vi "Wake up HL.vi"(6 "wait for reply (T)":bool=TRUE, 8 "error in":errorcluster, 10 "Acquisition data":T1, 11 "Module ID":i32=-1) -> (0 "error out":errorcluster, 1 "timed out?":bool, 3 "Data out":variant)   [LabVIEW 2020, in "NI DAQ.lvlib"]
doc: "Request to wake the helper loop to continuously read\\acquire from the specified task at a rate detemined by the timeout. Returns data as a variant.\n_____\nCreated using DQMH Event Scripter 6.1.0.128."
uses:
  NI DAQ.lvlib
  Support/Continuous aquisition params.ctl
  Support/Task list.ctl
  Wake up HL Argument--cluster.ctl
  Wake up HL (Reply Payload)--cluster.ctl
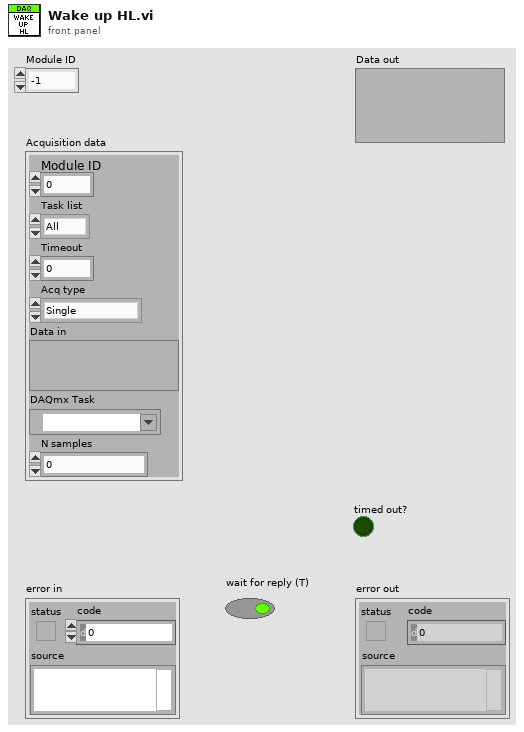
[diagram p1: front panel]
types:
  T1 = typedef "NI DAQ.lvlib/Continuous aquisition params.ctl" = cluster{"Module ID":i32, "Task list":T2, "Timeout":i32, "Acq type":enum16{"Single", "Multiple"}, "Data in":variant, "DAQmx Task":refnum<k21>, "N samples":i32}
  T2 = typedef "NI DAQ.lvlib/Task list.ctl" = enum16{"All", "DO task", "DI task", "AO task", "AI task"}
  T3 = typedef "NI DAQ.lvlib/Wake up HL Argument--cluster.ctl" = cluster{"Module ID":i32, "Wait Notifier":refnum<notifier>, "wait for reply":bool, "Acquisition data":T1}
  T4 = typedef "NI DAQ.lvlib/Request Events--cluster.ctl" = cluster{"Stop Module":refnum<user-event>, "Show Panel":refnum<user-event>, "Hide Panel":refnum<user-event>, "Show Diagram":refnum<user-event>, "Get Module Execution Status":refnum<user-event>, "Set device ID":refnum<user-event>, "Get channel list":refnum<user-event>, "Create DO task":refnum<user-event>, "Start task":refnum<user-event>, "Stop task":refnum<user-event>, "Write DO":refnum<user-event>, "Create DI channel":refnum<user-event>, "Read DI":refnum<user-event>, "Get task ref":refnum<user-event>, "Wake up HL":refnum<user-event>, "Sleep HL":refnum<user-event>, "Create AI channel":refnum<user-event>, "Read AI":refnum<user-event>, "Create AO channel":refnum<user-event>, "Write AO":refnum<user-event>, "Validate connection":refnum<user-event>, "Start continous acquisition":refnum<user-event>, "Stop continuous acquisition":refnum<user-event>}
  T5 = typedef "NI DAQ.lvlib/Wake up HL (Reply Payload)--cluster.ctl" = cluster{"data":variant, "error":errorcluster}
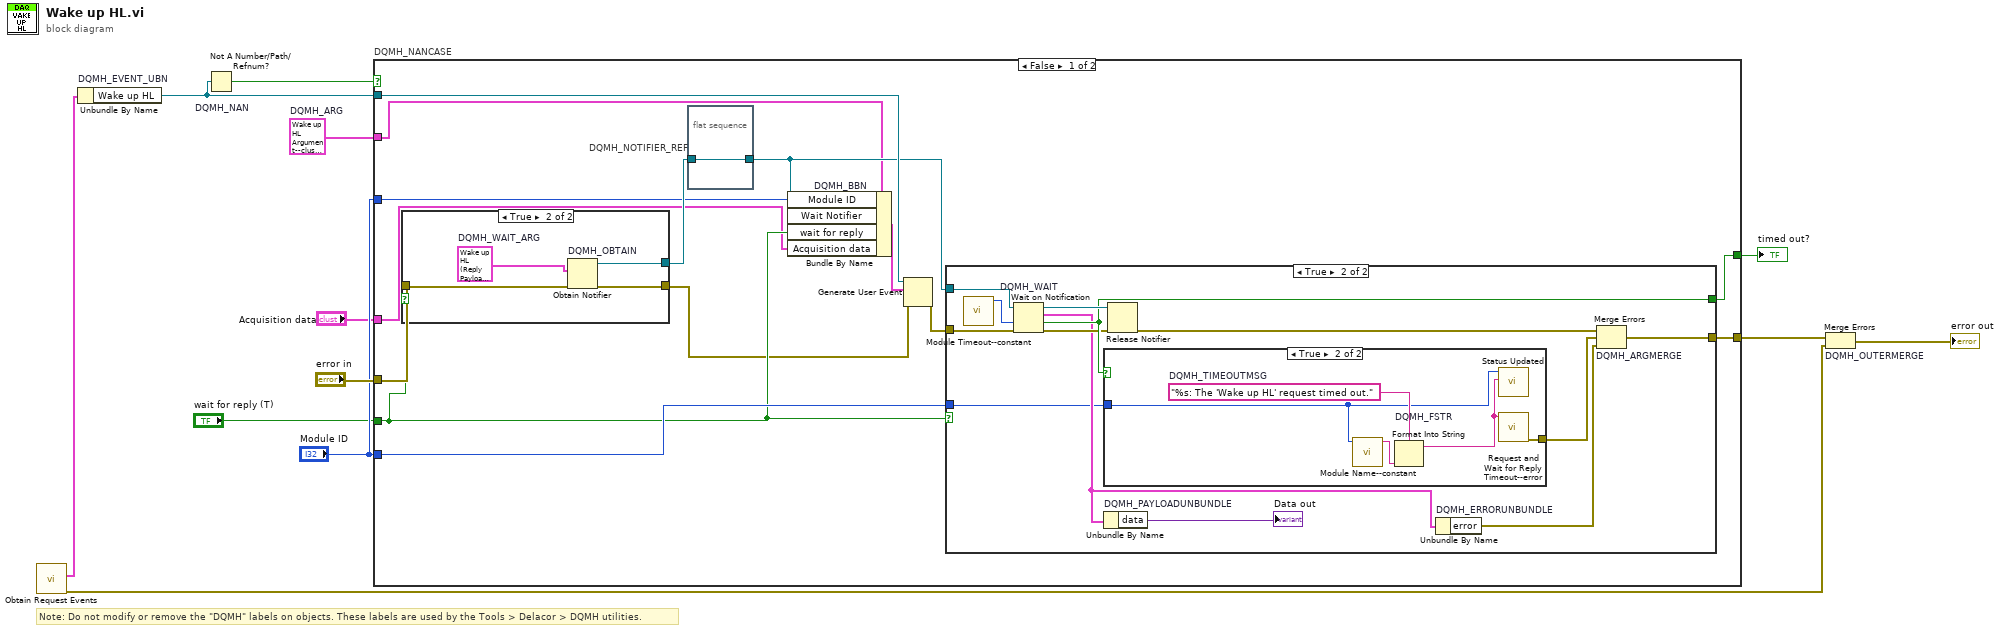
[diagram p0: block diagram]
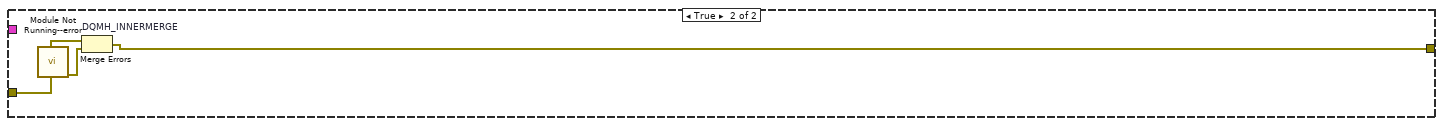
[diagram p5: hidden frame]
diagram:
  w6 = T3 {"Module ID"=-1, "Wait Notifier"=refnum, "wait for reply"=FALSE, "Acquisition data"={"Module ID"=0, "Task list"=enum."DO task", "Timeout"=0, "Acq type"=enum."Single", "Data in"=variant, "DAQmx Task"="", "N samples"=0}}  # DQMH_ARG
  # "Note: Do not modify or remove the \"DQMH\" labels on objects. These labels are used by the Tools > Delacor > DQMH utilities."
  n1 = call "Obtain Request Events.vi"() -> ("error out"=w3:errorcluster, "NI DAQ Request Events"=w2:T4)  [unwired: 10 in]
  n2 = Unbundle By Name "DQMH_EVENT_UBN"(w2) -> ("Wake up HL"=w10:refnum<user-event>)
  n3 = Not A Number/Path/Refnum? "DQMH_NAN"(number/path/refnum=w10) -> (NaN/Path/Refnum?=w9:bool)
  n4 = case "DQMH_NANCASE" shown="False" w9 {
    tunnel: "error in" -> [w26 w54]
    tunnel: w10 -> [w24 _]
    tunnel: [w22 w53] -> w7
    tunnel: [w23 _] -> w8
    tunnel: w6 -> [w18 _]
    tunnel: "Module ID" -> [w17 _]
    tunnel: "Module ID" -> [w16 _]
    tunnel: "wait for reply (T)" -> [w15 _]
    tunnel: "Acquisition data" -> [w13 _]
    frame False {
      n5 = case shown="True" w15 {
        tunnel: w26 -> [w47 w51]
        tunnel: [w47 w50] -> w14
        tunnel: [_ w48] -> w20
        frame False {
        }
        frame True {
          w49 = T5 {"data"=variant, "error"={"status"=FALSE, "code"=0, "source"=""}}  # DQMH_WAIT_ARG
          n6 = Obtain Notifier "DQMH_OBTAIN"(notification data type=w49, error in (no error)=w51) -> (notifier out=w48:refnum<notifier>, error out=w50:errorcluster)  [unwired: 2 in, 1 out]
        }
      }
      n7 = flat-sequence "DQMH_NOTIFIER_REF" {
        tunnel: w20 -> [w27]
        tunnel: [w27] -> w19
        frame #0 {
        }
      }
      n8 = Bundle By Name "DQMH_BBN"(cluster=w18, "Module ID"=w17, "Wait Notifier"=w19, "wait for reply"=w15, "Acquisition data"=w13) -> (w21:T3)
      n9 = Generate User Event(user event=w24, event data cluster=w21, error in=w14) -> (error out=w25:errorcluster)  [unwired: 1 in, 1 out]
      n10 = case shown="True" w15 {
        tunnel: w25 -> [w28 w41]
        tunnel: w19 -> [_ w40]
        tunnel: [_ w38] -> w23
        tunnel: [w28 w37] -> w22
        tunnel: w16 -> [_ w29]
        frame False {
        }
        frame True {
          n11 = call "Module Timeout--constant.vi"() -> ("Module Timeout"=w31:i32)  [unwired: 11 in]
          n12 = Wait on Notification "DQMH_WAIT"(notifier=w40, timeout in ms (-1)=w31, error in (no error)=w41) -> (notifier out=w39:refnum<notifier>, notification=w32:T5, timed out?=w38:bool, error out=w36:errorcluster)  [unwired: 1 in]
          n13 = case shown="True" w38 {
            tunnel: [_ w44] -> w33
            tunnel: w29 -> [_ w42]
            frame False {
            }
            frame True {
              w46 = "%s: The 'Wake up HL' request timed out."  # DQMH_TIMEOUTMSG
              n14 = call "Module Name--constant.vi"("Module ID"=w42) -> ("Module Name"=w43:string)  [unwired: 10 in]
              n15 = Format Into String "DQMH_FSTR"(format string=w46, w43) -> (resulting string=w45:string)  [unwired: 2 in, 1 out]
              n16 = call "Status Updated.vi"("Status"=w45, "Module ID"=w42) -> ()  [unwired: 9 in, 1 out]
              n17 = call "Request and Wait for Reply Timeout--error.vi"("Error Message"=w45) -> ("error out"=w44:errorcluster)  [unwired: 10 in]
            }
          }
          n18 = Unbundle By Name "DQMH_PAYLOADUNBUNDLE"(w32) -> ("data"=→"Data out":variant)
          n19 = Release Notifier(notifier=w39, error in (no error)=w36) -> (error out=w35:errorcluster)  [unwired: 1 in, 2 out]
          n20 = Unbundle By Name "DQMH_ERRORUNBUNDLE"(w32) -> ("error"=w34:errorcluster)
          n21 = Merge Errors "DQMH_ARGMERGE"(w35, w33, w34) -> (w37:errorcluster)
        }
      }
    }
    frame True {
      n22 = call "Module Not Running--error.vi"() -> ("error out"=w52:errorcluster)  [unwired: 11 in]
      n23 = Merge Errors "DQMH_INNERMERGE"(w54, w52) -> (w53:errorcluster)
    }
  }
  "timed out?" <- w8
  n24 = Merge Errors "DQMH_OUTERMERGE"(w7, w3) -> (→"error out":errorcluster)
